vi "LS Durability Main (FPGA).vi"() -> ()   [LabVIEW 2018]
uses:
  <vilib>/rvi/Emulation/niFpgaGetClockAttributes.vi
  <vilib>/rvi/Emulation/niFpgaSctlEmulationGetInTimedLoop.vi
  <vilib>/rvi/Emulation/niFpgaEmulationReportErrorSimple.vi
  <vilib>/rvi/Emulation/niFpgaProcessEmulError.vi
  <vilib>/rvi/eio/common/nirviEmuTemplateMethod_errors.vi
  <vilib>/rvi/Emulation/niFpgaCriticalErrorInLSC.vi
  <vilib>/rvi/DataTransferAndStorage/Container/Common/niFpgaContainerExecOnDevCompGetState.vi
  <vilib>/rvi/Emulation/niFpgaEmulationIsFPGAContextNoSignature.vi
  <vilib>/rvi/errors/niFpgaSetErrorForExecOnDevCompSimple.vi
  <vilib>/rvi/eio/common/nirviEmuReportErrorAndStop.vi
  <vilib>/rvi/DataTransferAndStorage/Container/Common/niFpgaContainerGetUniqueNameForEmu.vi
  <vilib>/rvi/FIFO/Fifo_Resource/nirvififoEmulationSetSize.vi
  <vilib>/rvi/FIFO/Fifo_Resource/nirviFifoEmulationQueueMgr.vi
  <instcachedir>/0/nirviFifoEmulationQueueMgr_E5CAEC123FF24DC58D834DCA3CDAA9B5.lvgen/nirviFifoEmulationQueueMgr_E5CAEC123FF24DC58D834DCA3CDAA9B5_003.vi
  <vilib>/rvi/FIFO/Fifo_Resource/nirvififoEmulationDetermineInputValidOut.vi
  <vilib>/rvi/FIFO/Fifo_Resource/nirvififoEmulationCreateLock.vi
  <vilib>/rvi/FIFO/Fifo_Resource/nirvififoEmulationObtainLock.vi
  <vilib>/rvi/FIFO/Fifo_Resource/nirvififoEmulationReleaseLock.vi
  <vilib>/rvi/occurrence/nirviWaitOnOccurrenceBase.vi
  <vilib>/rvi/errors/nirviReportUnexpectedCaseInternalError.vi
  <vilib>/rvi/errors/nirviReportUnexpectedCaseInternalError (U32).vi
  <vilib>/Utility/error.llb/Clear Errors.vi
  <vilib>/rvi/interface/RandomDataEmulation/niFpgaRandomDataHandleErrors.vi
  <vilib>/eio/EIONode/EIONode.xnode
  <vilib>/rvi/FXPMathLib/FxpAdd/XNode/nifxpmath_Add.xnode
  <vilib>/rvi/DataTransferAndStorage/Container/XNode/niFpgaContainer.xnode
  <vilib>/rvi/FIFO/Fifo_Resource/niFpgaFifoEmulationRefIn.vi
  <vilib>/rvi/FXPMathLib/sim/FxpSim.dll
panel:
  in  "B2offset":fxp<+/-,24,5>
  in  "B1offset":fxp<+/-,24,5>
  out "FIFO microseconds":u32
  in  "V(T)/R(F)":bool=TRUE
  in  "Resistance In":fxp<+/-,28,17>[](array[numeric])=[0.0, 0.0, 0.0, 0.0, 0.0, 0.0, 0.0, 0.0, 0.0, 0.0, 0.0, 0.0]
  out "Anomaly Resamples":fxp<+/-,28,17>[](array[numeric])
  in  "Anomaly Threshold":fxp<+/-,28,17>=0.02978515625
  out "Bank2Active":bool
  out "Bank1Active":bool
  out "Bank2On":bool
  out "Bank1On":bool
  in  "Enable Readings":bool[](array[boolean])=[FALSE, FALSE, FALSE, FALSE, FALSE, FALSE, FALSE, FALSE, FALSE, FALSE, FALSE, FALSE]
  in  "Opens Resets":bool[](array[boolean])=[FALSE, FALSE, FALSE, FALSE, FALSE, FALSE, FALSE, FALSE, FALSE, FALSE, FALSE, FALSE]
  in  "Enable Opens":bool[](array[boolean])=[FALSE, FALSE, FALSE, FALSE, FALSE, FALSE, FALSE, FALSE, FALSE, FALSE, FALSE, FALSE]
  out "Opens Detected":u16[](array[numeric])
  out "Opens Loop Time (usec)":u32=1000
  in  "Bank2(Pulse/Const)":bool
  in  "Bank2Const(On/Off)":bool
  out "Anomalies (Last Cycle)":i32[](array[numeric])
  out "Cycle Starts":bool[](array[boolean])
  out "Anomalies (Total)":i32[](array[numeric])
  out "Anomalies/Cycle":i32[](array[numeric])
  in  "Normal Steps":u32=98
  out "Cycles":u32[](array[numeric])
  out "Anomaly Loop Time (usec)":u32=1000
  out "Steps":u32[](array[numeric])
  in  "Step Threshold":fxp<+/-,28,17>=0.02978515625
  in  "Enable Anomalies":bool[](array[boolean])=[FALSE, FALSE, FALSE, FALSE, FALSE, FALSE, FALSE, FALSE, FALSE, FALSE, FALSE, FALSE]
  in  "Anomaly Resets":bool[](array[boolean])=[FALSE, FALSE, FALSE, FALSE, FALSE, FALSE, FALSE, FALSE, FALSE, FALSE, FALSE, FALSE]
  in  "Bank1Const(On/Off)":bool
  in  "Bank1(Pulse/Const)":bool
  in  "PWM Period (Ticks)":u32=4000000
  in  "Duty (Ticks)":i32=2000000
  in  "Invert PWM?":bool=TRUE
  in  "Cycle Resets":bool[](array[boolean])=[FALSE, FALSE, FALSE, FALSE, FALSE, FALSE, FALSE, FALSE, FALSE, FALSE, FALSE, FALSE]
  in  "Points to Avg":i32=20
  in  "Enable Cycles":bool[](array[boolean])=[FALSE, FALSE, FALSE, FALSE, FALSE, FALSE, FALSE, FALSE, FALSE, FALSE, FALSE, FALSE]
  out "Total Cycles":u32[](array[numeric])
  in  "Cycle Threshold":fxp<+/-,28,17>=1.2001953125
  out "Analog Inputs":fxp<+/-,28,17>[](array[numeric])
  out "AI Loop Time (usec)":u32=70
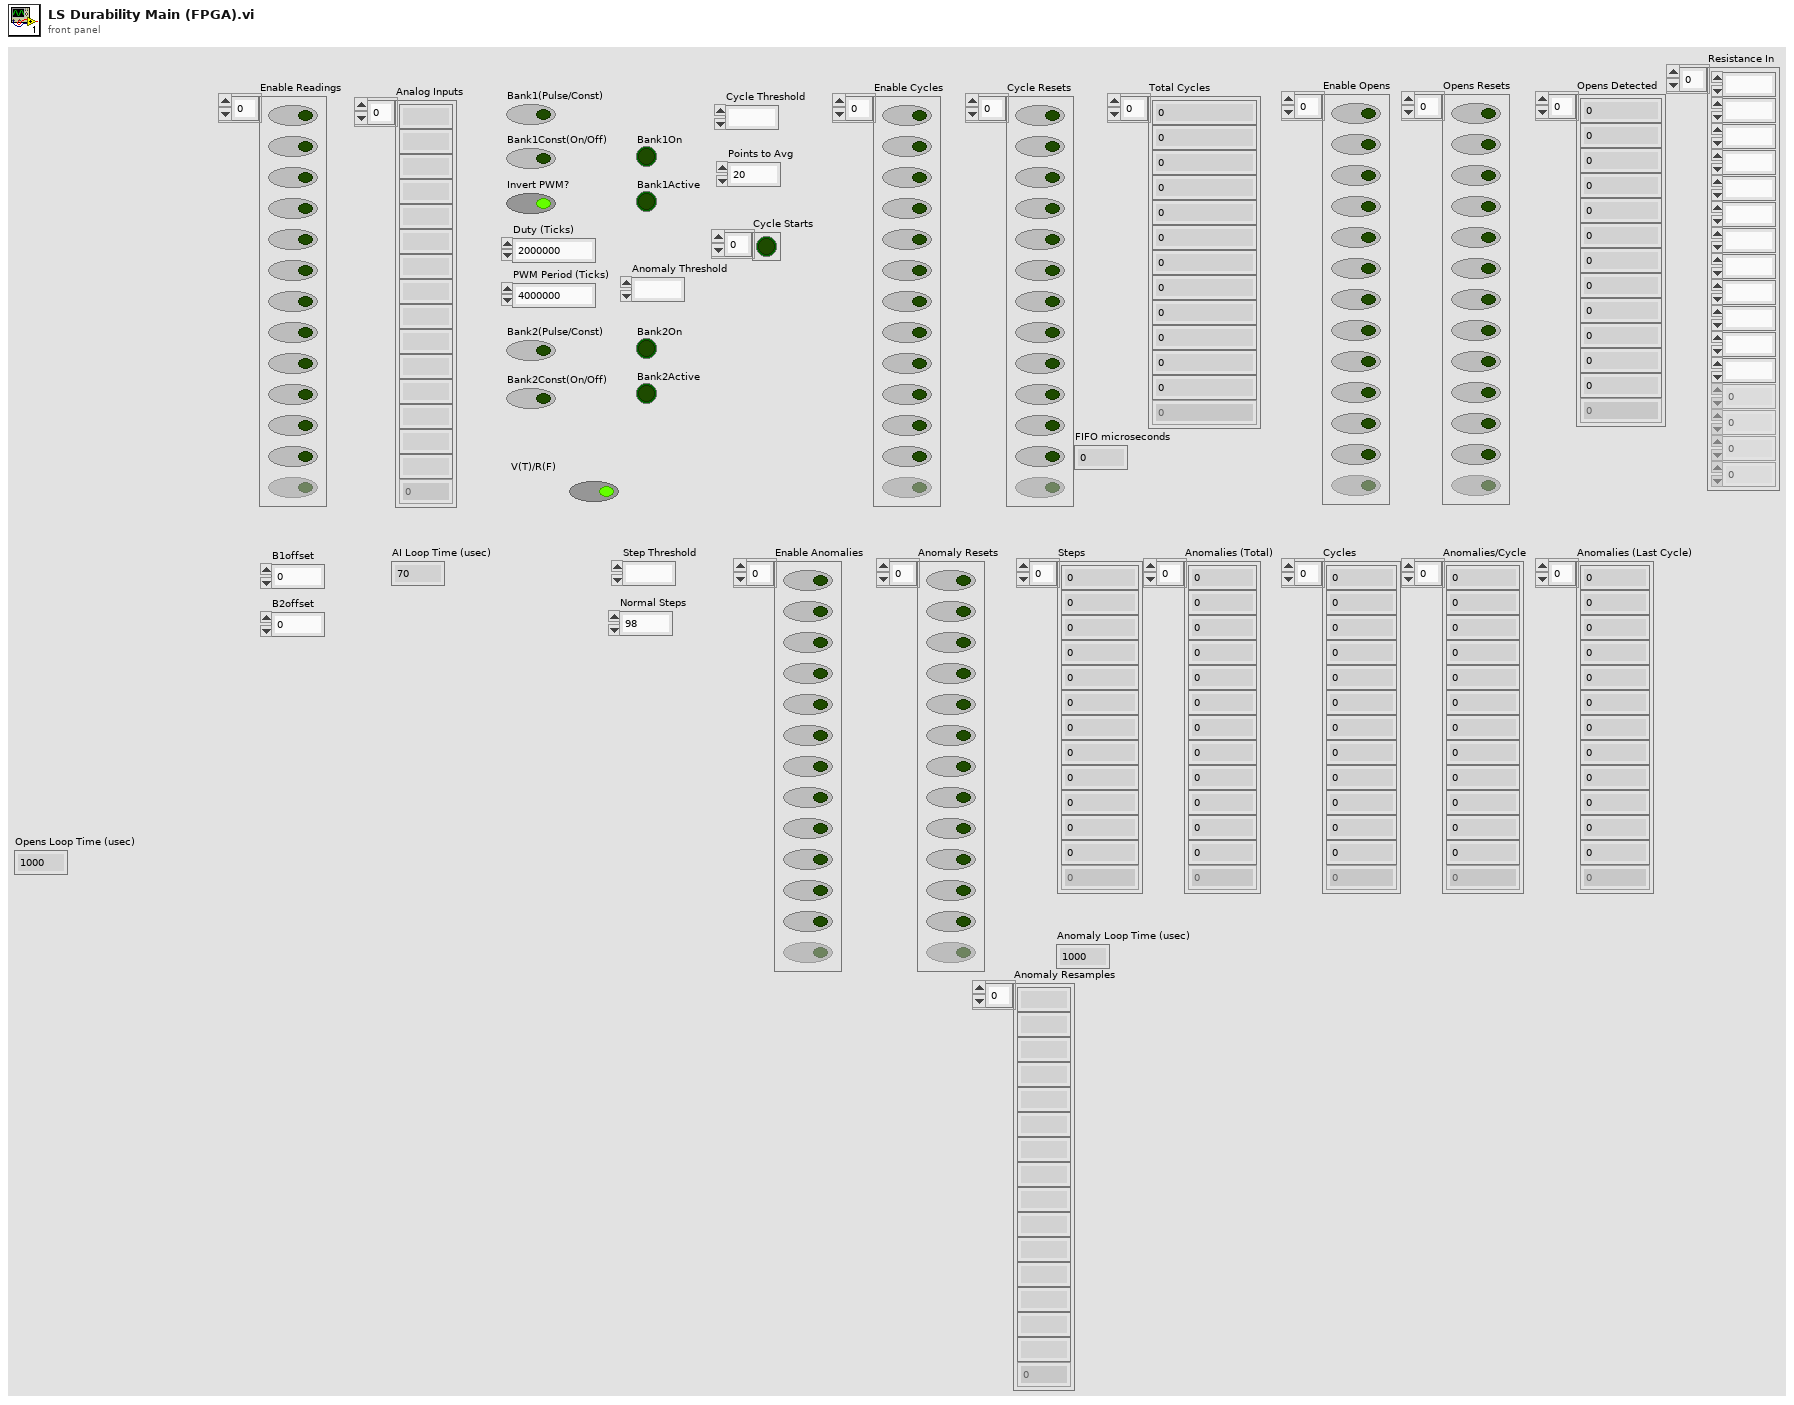
[diagram p1: front panel]
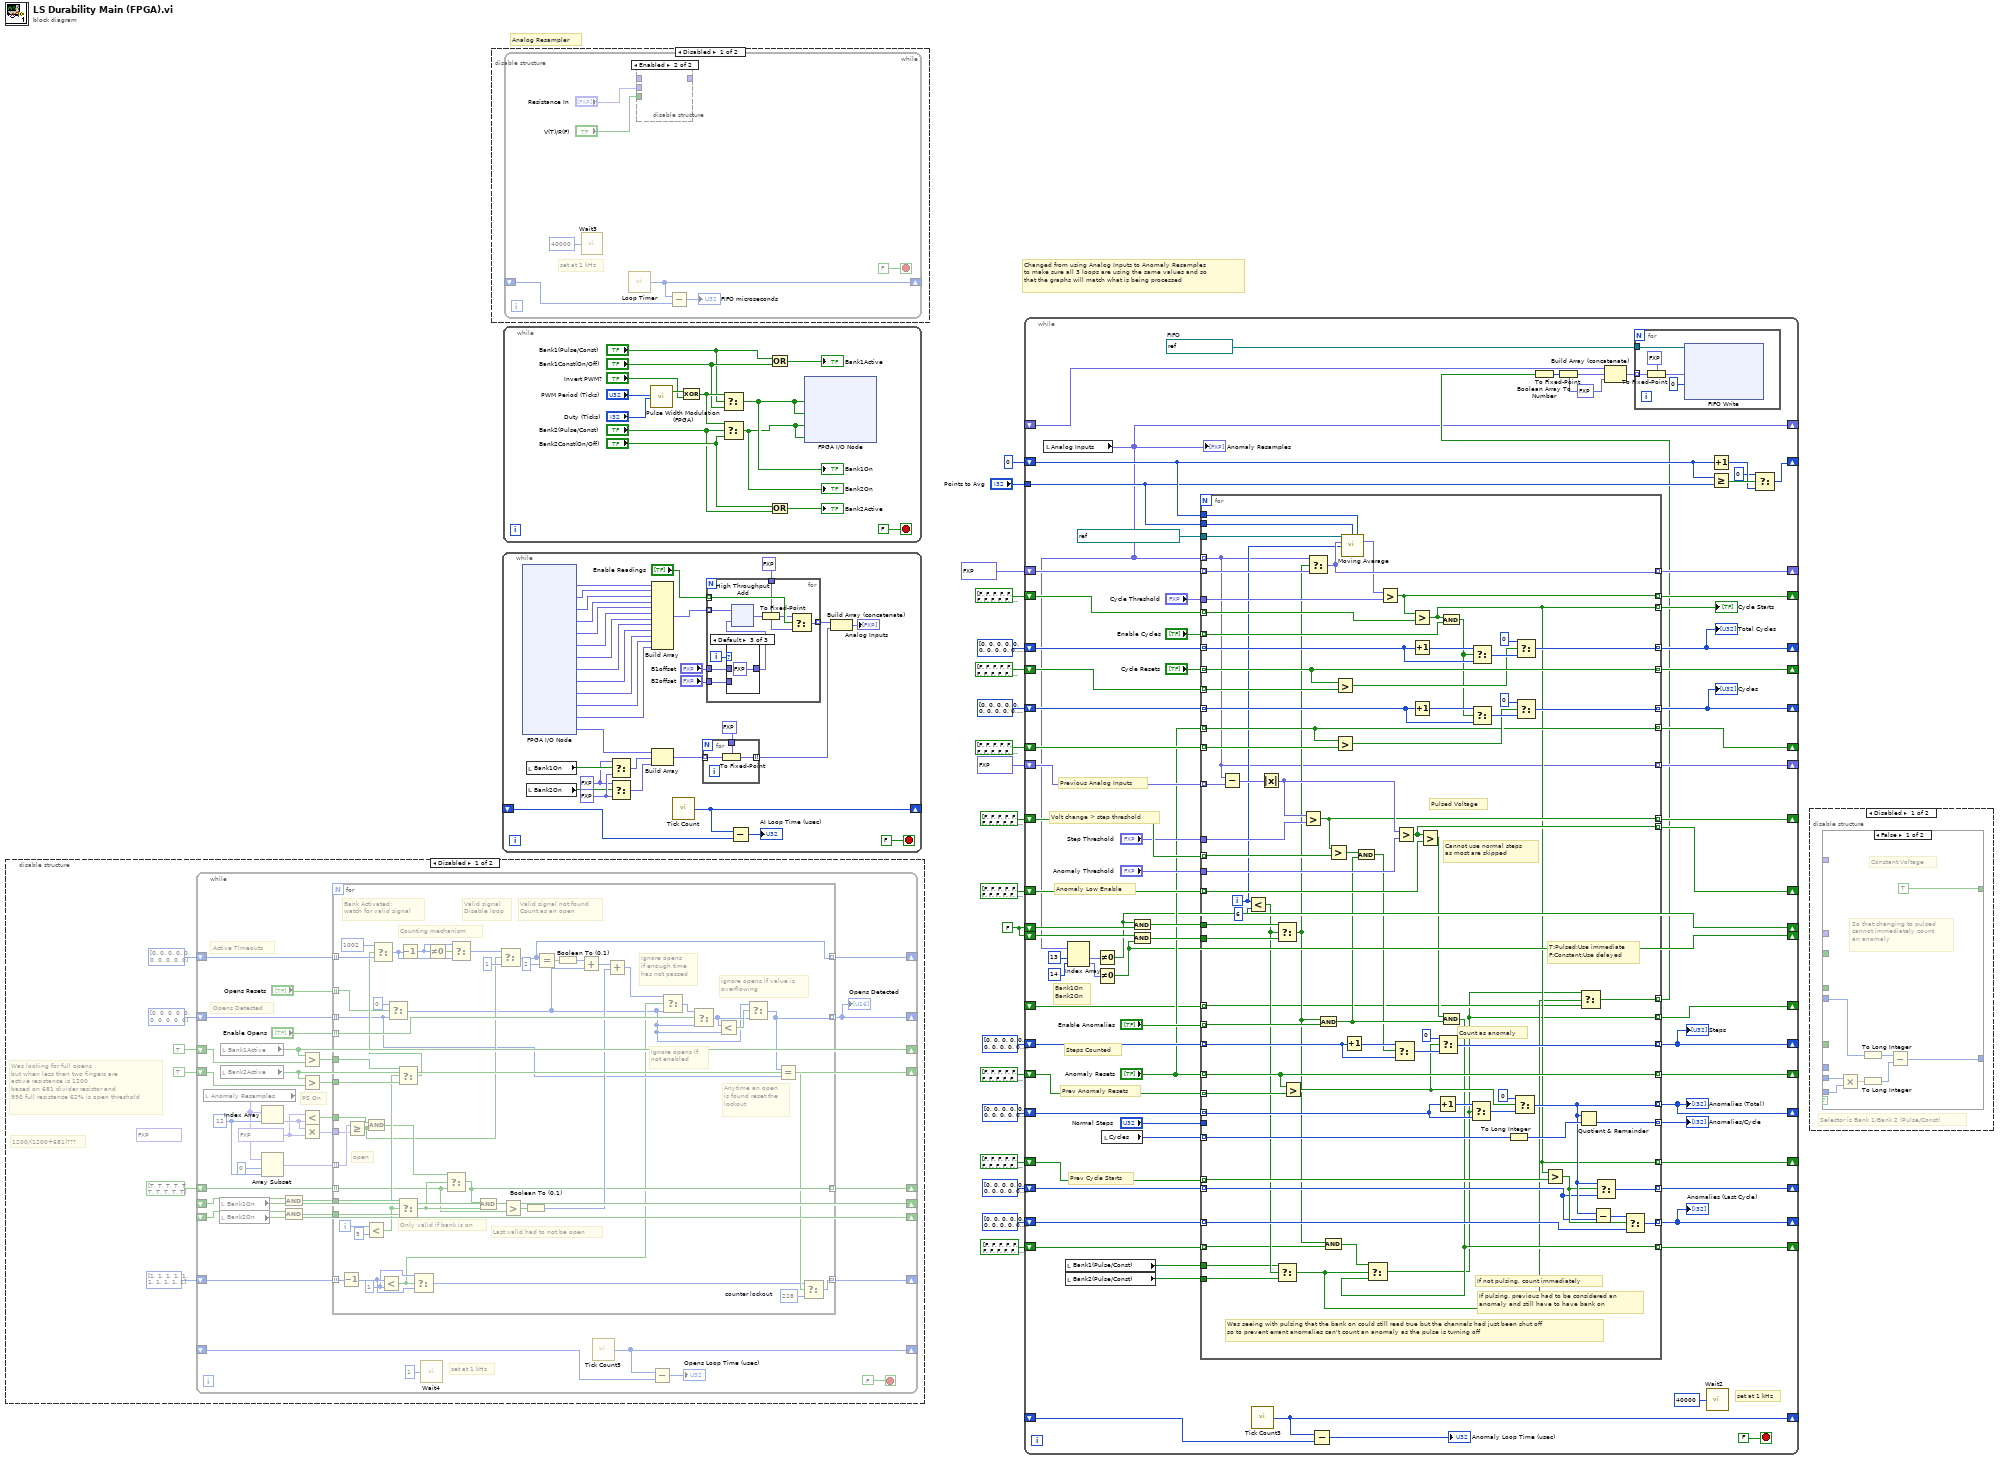
[diagram p0: block diagram]
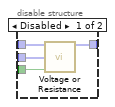
[diagram p2: hidden frame]
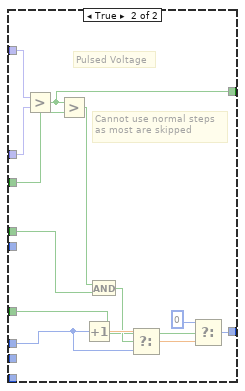
[diagram p5: hidden frame]
diagram:
  w2 = FALSE
  # "Changed from using Analog Inputs to Anomaly Resamples\nto make sure all 3 loops are using the same values and so\nthat the graphs will match what is being processed"
  # "Analog Resampler"
  n1 = disable-structure shown="Disabled" {
    frame Disabled {
      (unwired) fxp<+,8,0> 0.94921875
      # "1200/(1200+681)???"
      # "Was looking for full opens\nbut when less than two fingers are\nactive resistance is 1200\nbased on 681 divider resistor and\n990 full resistance 62% is open threshold"
      n2 = while {
        shift-right: [w58] -> _
        shift-left: _ -> [w57]
        shift-right: [w29] -> _
        shift-left: u8[] [0, 0, 0, 0, 0, 0, 0, 0, 0, 0] -> [w53]
        shift-right: [w38] -> _
        shift-left: u16[] [0, 0, 0, 0, 0, 0, 0, 0, 0, 0] -> [w39]
        shift-right: [w45] -> _
        shift-left: bool[] [TRUE, TRUE, TRUE, TRUE, TRUE, TRUE, TRUE, TRUE, TRUE, TRUE] -> [w44]
        shift-right: [w43] -> _
        shift-left: TRUE ("Bank2Active") -> [w41]
        shift-right: [w42] -> _
        shift-left: TRUE ("Bank1Active") -> [w40]
        shift-right: [w32] -> _
        shift-left: _ -> [w30]
        shift-right: [w33] -> _
        shift-left: _ -> [w31]
        shift-right: [w27] -> _
        shift-left: u16[] [1, 1, 1, 1, 1, 1, 1, 1, 1, 1] -> [w28]
        stop <- FALSE stop-if-true
        w46 = fxp<+,8,0> 0.62109375
        w55 = 12 ("length")
        # "Opens Detected"
        # "Active Timeouts"
        # "PS On"
        # "set at 1 kHz"
        n3 = local read "Anomaly Resamples"() -> (w26:fxp<+/-,28,17>[])
        n4 = local read "Bank1On"() -> (w33:bool)
        n5 = local read "Bank2On"() -> (w32:bool)
        n6 = local read "Bank1Active"() -> (w42:bool)
        n7 = local read "Bank2Active"() -> (w43:bool)
        n8 = Index Array(array=w26, index=w55) -> (element=w47:fxp<+/-,28,17>)
        n9 = Array Subset(array=w26, index=0, length=w55) -> (w48:fxp<+/-,28,17>[])
        n10 = And(x=w31, y=w33) -> (x .and. y?=w35:bool)
        n11 = And(x=w30, y=w32) -> (x .and. y?=w34:bool)
        n12 = Greater?(x=w42, y=w40) -> (0:w52:bool)
        n13 = Greater?(x=w43, y=w41) -> (0:w51:bool)
        n14 = Less?(x=w46, y=w47) -> (x < y?=w50:bool)
        n15 = Multiply(x=w47, y=w46) -> (x*y=w49:fxp<+/-,36,17>)
        n16 = for {
          tunnel: w35 -> [w107]
          tunnel: w34 -> [w106]
          tunnel: w52 -> [w104]
          tunnel: w51 -> [w105]
          tunnel: w53 -> [w65] mode=indexing
          tunnel: w39 -> [w92] mode=indexing
          tunnel: "Opens Resets" -> [w76] mode=indexing
          tunnel: "Enable Opens" -> [w90] mode=indexing
          tunnel: [w66] -> w29 mode=indexing
          tunnel: w49 -> [w87]
          tunnel: w48 -> [w88] mode=indexing
          tunnel: w50 -> [w86]
          tunnel: [w77] -> w45 mode=indexing
          tunnel: w44 -> [w82] mode=indexing
          tunnel: [w80] -> w38 mode=indexing
          tunnel: w28 -> [w71] mode=indexing
          tunnel: [w67] -> w27 mode=indexing
          i -> [w109]
          w68 = u16 228  # counter lockout
          w72 = u16 1 ("y")
          # "Ignore opens if\nnot enabled"
          # "Ignore opens\nif enough time\nhas not passed"
          # "Anytime an open\nis found reset the\nlockout"
          # "ignore opens if value is\noverflowing"
          # "Last valid had to not be open"
          # "Only valid if bank is on"
          # "open"
          # "Valid signal not found\nCount as an open"
          # "Valid signal\nDisable loop"
          # "Counting mechanism"
          # "Bank Activated:\nwatch for valid signal"
          n17 = Decrement(x=w71) -> (x-1=w73:u16)
          n18 = Greater Or Equal?(x=w88, y=w87) -> (x >= y?=w79:bool)
          n19 = Less?(x=w109, y=5) -> (x < y?=w103:bool)
          n20 = And(x=w86, y=w79) -> (x .and. y?=w85:bool)
          n21 = Less?(x=w73, y=w72) -> (x < y?=w62:bool)
          n22 = Select(t=u16 0, s=w76, f=w65) -> (s? t:f=w61:u16)
          n23 = Select(t=w104, s=w103, f=w105) -> (s? t:f=w89:bool)
          n24 = Select(t=u16 1002, s=w89, f=w92) -> (s? t:f=w91:u16)
          n25 = Select(t=w107, s=w103, f=w106) -> (s? t:f=w84:bool)
          n26 = Decrement(x=w91) -> (x-1=w96:u16)
          n27 = Select(t=w72, s=w62, f=w73) -> (s? t:f=w69:u16)
          n28 = Not Equal To 0?(x=w96) -> (x != 0?=w95:bool)
          n29 = Select(t=w85, s=w84, f=w82) -> (s? t:f=w77:bool)
          n30 = Select(t=w96, s=w95, f=w91) -> (s? t:f=w97:u16)
          n31 = And(x=w77, y=w84) -> (x .and. y?=w78:bool)
          n32 = Select(t=w97, s=w79, f=u16 1) -> (s? t:f=w80:u16)
          n33 = Greater?(x=w78, y=w82) -> (0:w83:bool)
          n34 = Boolean To (0,1)(Boolean=w83) -> (0, 1=w81:i16)
          n35 = Equal?(x=w80, y=u16 2) -> (x = y?=w99:bool)
          n36 = Boolean To (0,1)(Boolean=w99) -> (0, 1=w100:i16)
          n37 = Add(x=w100, y=w61) -> (x+y=w101:u16)
          n38 = Add(x=w101, y=w81) -> (x+y=w63:u16)
          n39 = Select(t=w63, s=w62, f=w61) -> (s? t:f=w64:u16)
          n40 = Select(t=w64, s=w90, f=w61) -> (s? t:f=w74:u16)
          n41 = Less?(x=w74, y=w61) -> (x < y?=w75:bool)
          n42 = Select(t=w61, s=w75, f=w74) -> (s? t:f=w66:u16)
          n43 = Equal?(x=w66, y=w65) -> (x = y?=w70:bool)
          n44 = Select(t=w69, s=w70, f=w68) -> (s? t:f=w67:u16)
        }
        "Opens Detected" <- w29
        n45 = call "Wait4"("Count(mSec)"=u32 1) -> ()  [unwired: 1 out]
        n46 = call "Tick Count5"() -> ("Tick Count(uSec)"=w58:u32)
        n47 = Subtract(x=w58, y=w57) -> (x-y=→"Opens Loop Time (usec)":u32)
      }
    }
    frame Enabled {
    }
  }
  n48 = disable-structure shown="Disabled" {
    frame Disabled {
      n49 = while {
        shift-right: [w111] -> _
        shift-left: _ -> [w112]
        stop <- FALSE stop-if-true
        # "set at 1 kHz"
        n50 = call "Wait3"("Count(Ticks)"=u32 40000 ("Count(mSec)")) -> ()  [unwired: 1 out]
        n51 = call "Loop Timer"() -> ("Tick Count(uSec)"=w111:u32)  [unwired: 1 in]
        n52 = disable-structure shown="Enabled" {
          disable-tunnel: _ -> [w120 _]
          disable-tunnel: [w119 _] -> _
          disable-tunnel: "Resistance In" -> [w118 _]
          disable-tunnel: "V(T)/R(F)" -> [w117 _]
          frame Disabled {
            n53 = call "Voltage or Resistance.vi"("Data In"=w120, "Resistance In"=w118, "V(T)/R(F)"=w117) -> ("Data Out"=w119:fxp<+/-,28,17>[])  [unwired: 12 in]
          }
          frame Enabled {
          }
        }
        n54 = Subtract(x=w111, y=w112) -> (x-y=→"FIFO microseconds":u32)
      }
    }
    frame Enabled {
    }
  }
  n55 = while {
    shift-right: [w152] -> _
    shift-left: _ -> [w151]
    stop <- FALSE stop-if-true
    w128 = fxp<+/-,24,5> 1.0 ("AI13")
    w131 = fxp<+/-,24,5> 0.0 ("AI13")
    n56 = xnode "FPGA I/O Node"() -> ("AI0"=w149:fxp<+/-,24,5>, "AI1"=w148:fxp<+/-,24,5>, "AI2"=w147:fxp<+/-,24,5>, "AI3"=w146:fxp<+/-,24,5>, "AI4"=w145:fxp<+/-,24,5>, "AI5"=w121:fxp<+/-,24,5>, "AI6"=w144:fxp<+/-,24,5>, "AI7"=w143:fxp<+/-,24,5>, "AI8"=w142:fxp<+/-,24,5>, "AI9"=w141:fxp<+/-,24,5>, "AI10"=w123:fxp<+/-,24,5>, "AI11"=w122:fxp<+/-,24,5>, "AI12"=w138:fxp<+/-,24,5>)  [unwired: 13 in, 13 out]
    n57 = local read "Bank1On"() -> (w130:bool)
    n58 = local read "Bank2On"() -> (w129:bool)
    n59 = Select(t=w128, s=w130, f=w131) -> (s? t:f=w127:fxp<+/-,24,5>)
    n60 = Select(t=w128, s=w129, f=w131) -> (s? t:f=w126:fxp<+/-,24,5>)
    n61 = Build Array(w149, w148, w147, w146, w145, w121, w144, w143, w142, w141, w123, w122) -> (w140:fxp<+/-,24,5>[])
    n62 = Build Array(w138, w127, w126) -> (w136:fxp<+/-,24,5>[])
    n63 = call "Tick Count"() -> ("Tick Count(uSec)"=w152:u32)
    n64 = for {
      tunnel: w136 -> [w156] mode=indexing
      tunnel: fxp<+/-,28,17> 0.0 ("AI0") -> [w155]
      tunnel: [w154] -> w135 mode=indexing
      n65 = To Fixed-Point(fixed-point type=w155, number=w156) -> (fixed-point=w154:fxp<+/-,28,17>)
    }
    n66 = for {
      tunnel: w140 -> [w159] mode=indexing
      tunnel: fxp<+/-,28,17> 0.0 ("AI0") -> [w164]
      tunnel: [w163] -> w134 mode=indexing
      tunnel: "Enable Readings" -> [w166] mode=indexing
      tunnel: "B1offset" -> [w161]
      tunnel: "B2offset" -> [w160]
      i -> [w162]
      n67 = case shown="Default" w162 {
        tunnel: w161 -> [w167 _ _]
        tunnel: w160 -> [_ w168 _]
        tunnel: [w167 w168 fxp<+/-,24,5> 0.0 ("B2offset")] -> w158
        frame 0..4 {
        }
        frame 5..9 {
        }
        frame Default {
        }
      }
      n68 = xnode "High Throughput Add"("x"=w159, "y"=w158) -> ("x+y"=w157:fxp<+/-,25,6>)
      n69 = To Fixed-Point(fixed-point type=w164, number=w157) -> (fixed-point=w165:fxp<+/-,28,17>)
      n70 = Select(t=w165, s=w166, f=w164) -> (s? t:f=w163:fxp<+/-,28,17>)
    }
    n71 = Subtract(x=w152, y=w151) -> (x-y=→"AI Loop Time (usec)":u32)
    n72 = Build Array (concatenate)(w134, w135) -> (→"Analog Inputs":fxp<+/-,28,17>[])
  }
  n73 = while {
    stop <- FALSE stop-if-true
    n74 = call "Pulse Width Modulation (FPGA).vi"("PWM Period (Ticks)"="PWM Period (Ticks)", "PWM Duty Cycle (Ticks)"="Duty (Ticks)") -> ("PWM DO"=w180:bool)  [unwired: 14 in, 3 out]
    n75 = Exclusive Or(1:"Invert PWM?", 2:w180) -> (0:w178:bool)
    n76 = Select(t=w178, s="Bank1(Pulse/Const)", f="Bank1Const(On/Off)") -> (s? t:f=w171:bool)
    "Bank1On" <- w171
    n77 = Select(t=w178, s="Bank2(Pulse/Const)", f="Bank2Const(On/Off)") -> (s? t:f=w170:bool)
    "Bank2On" <- w170
    n78 = Or(x="Bank1(Pulse/Const)", y="Bank1Const(On/Off)") -> (x .or. y?=→"Bank1Active":bool)
    n79 = Or(x="Bank2Const(On/Off)", y="Bank2(Pulse/Const)") -> (x .or. y?=→"Bank2Active":bool)
    n80 = xnode "FPGA I/O Node"("RMC/DIO0"=w171, "DIO0"=w171, "RMC/DIO1"=w170, "DIO1"=w170) -> ()  [unwired: 5 in, 5 out]
  }
  n81 = while {
    shift-right: [w257] -> _
    shift-left: _ -> [w256]
    shift-right: [w250] -> _
    shift-left: bool[] [FALSE, FALSE, FALSE, FALSE, FALSE, FALSE, FALSE, FALSE, FALSE, FALSE, FALSE, FALSE] -> [w249]
    shift-right: [w247] -> _
    shift-left: u32[] [0, 0, 0, 0, 0, 0, 0, 0, 0, 0, 0, 0] -> [w246]
    shift-right: [w245] -> _
    shift-left: bool[] [FALSE, FALSE, FALSE, FALSE, FALSE, FALSE, FALSE, FALSE, FALSE, FALSE, FALSE, FALSE] -> [w243]
    shift-right: [w252] -> _
    shift-left: fxp<+/-,28,17>[] [0.0, 0.0, 0.0, 0.0, 0.0, 0.0, 0.0, 0.0, 0.0, 0.0, 0.0, 0.0] -> [w251]
    shift-right: [w241] -> _
    shift-left: bool[] [FALSE, FALSE, FALSE, FALSE, FALSE, FALSE, FALSE, FALSE, FALSE, FALSE, FALSE, FALSE] -> [w240]
    shift-right: [w239] -> _
    shift-left: i32[] [0, 0, 0, 0, 0, 0, 0, 0, 0, 0, 0, 0] -> [w237]
    shift-right: [w238] -> _
    shift-left: i32[] [0, 0, 0, 0, 0, 0, 0, 0, 0, 0, 0, 0] -> [w236]
    shift-right: [w193] -> _
    shift-right: [w194] -> _
    shift-right: [w235] -> _
    shift-left: i32[] [0, 0, 0, 0, 0, 0, 0, 0, 0, 0, 0, 0] -> [w234]
    shift-right: [w231] -> _
    shift-left: bool[] [FALSE, FALSE, FALSE, FALSE, FALSE, FALSE, FALSE, FALSE, FALSE, FALSE, FALSE, FALSE] -> [w232]
    shift-left: w2 -> [w229]
    shift-left: w2 -> [w230]
    tunnel: "Points to Avg" -> [w204]
    shift-right: [w224] -> _
    shift-left: 0 ("Moving Point Index") -> [w205]
    shift-right: [w206] -> _
    shift-left: fxp<+/-,28,17>[] [0.0, 0.0, 0.0, 0.0, 0.0, 0.0, 0.0, 0.0, 0.0, 0.0, 0.0, 0.0] ("Analog Inputs") -> [w208]
    shift-right: [w209] -> _
    shift-left: bool[] [FALSE, FALSE, FALSE, FALSE, FALSE, FALSE, FALSE, FALSE, FALSE, FALSE, FALSE, FALSE] -> [w211]
    shift-right: [w214] -> _
    shift-left: u32[] [0, 0, 0, 0, 0, 0, 0, 0, 0, 0, 0, 0] -> [w215]
    shift-right: [w216] -> _
    shift-left: bool[] [FALSE, FALSE, FALSE, FALSE, FALSE, FALSE, FALSE, FALSE, FALSE, FALSE, FALSE, FALSE] -> [w218]
    shift-right: [w220] -> _
    shift-left: u32[] [0, 0, 0, 0, 0, 0, 0, 0, 0, 0, 0, 0] -> [w221]
    shift-right: [w219] -> _
    shift-left: bool[] [FALSE, FALSE, FALSE, FALSE, FALSE, FALSE, FALSE, FALSE, FALSE, FALSE, FALSE, FALSE] -> [w223]
    shift-right: [w200] -> _
    shift-left: bool[] [FALSE, FALSE, FALSE, FALSE, FALSE, FALSE, FALSE, FALSE, FALSE, FALSE, FALSE, FALSE] -> [w199]
    shift-right: [w184] -> _
    shift-left: _ -> [w188]
    shift-right: [w186] -> _
    shift-left: _ -> [w187]
    stop <- FALSE stop-if-true
    w189 = refnum<k21> "Analog Data"  # FIFO
    w191 = fxp<+/-,28,17> -15.0 ("AI0")
    # "Bank1On\nBank2On"
    # "Anomaly Low Enable"
    # "Prev Cycle Starts"
    # "Prev Anomaly Resets"
    # "Steps Counted"
    # "Volt change > step threshold"
    # "Previous Analog Inputs"
    # "set at 1 kHz"
    n82 = local read "Analog Inputs"() -> (w184:fxp<+/-,28,17>[])
    "Anomaly Resamples" <- w184
    n83 = local read "Bank1(Pulse/Const)"() -> (w202:bool)
    n84 = local read "Bank2(Pulse/Const)"() -> (w201:bool)
    n85 = Index Array(array=w184, index #1=13 ("index"), index #2=14 ("index")) -> (element #1=w196:fxp<+/-,28,17>, element #2=w195:fxp<+/-,28,17>)
    n86 = Not Equal To 0?(x=w196) -> (x != 0?=w193:bool)
    n87 = Not Equal To 0?(x=w195) -> (x != 0?=w194:bool)
    n88 = local read "Cycles"() -> (w242:u32[])
    n89 = And(x=w193, y=w230) -> (x .and. y?=w254:bool)
    n90 = And(x=w229, y=w194) -> (x .and. y?=w253:bool)
    n91 = for {
      tunnel: [w309] -> w250 mode=indexing
      tunnel: w249 -> [w324] mode=indexing
      tunnel: w246 -> [w318] mode=indexing
      tunnel: [w317] -> w247 mode=indexing
      tunnel: "Step Threshold" -> [w310]
      tunnel: "Enable Anomalies" -> [w280] mode=indexing
      tunnel: "Anomaly Resets" -> [w326] mode=indexing
      tunnel: [w326] -> w245 mode=indexing
      tunnel: w243 -> [w327] mode=indexing
      tunnel: [w270] -> w252 mode=indexing
      tunnel: w251 -> [w341] mode=indexing
      tunnel: "Normal Steps" -> [_]
      tunnel: w242 -> [w333] mode=indexing
      tunnel: [w332] -> w244 mode=indexing
      tunnel: [w334] -> w235 mode=indexing
      tunnel: [w278] -> w241 mode=indexing
      tunnel: w240 -> [w329] mode=indexing
      tunnel: [w331] -> w239 mode=indexing
      tunnel: w237 -> [w316] mode=indexing
      tunnel: [w330] -> w238 mode=indexing
      tunnel: w236 -> [w315] mode=indexing
      tunnel: w254 -> [w346]
      tunnel: w253 -> [w345]
      tunnel: w234 -> [w343] mode=indexing
      tunnel: "Anomaly Threshold" -> [w339]
      tunnel: w232 -> [w338] mode=indexing
      tunnel: [w337] -> w231 mode=indexing
      tunnel: w223 -> [w308] mode=indexing
      tunnel: "Anomaly Resets" -> [w301] mode=indexing
      tunnel: w221 -> [w304] mode=indexing
      tunnel: [w303] -> w220 mode=indexing
      tunnel: [w301] -> w219 mode=indexing
      tunnel: w218 -> [w300] mode=indexing
      tunnel: "Cycle Resets" -> [w299] mode=indexing
      tunnel: [w299] -> w216 mode=indexing
      tunnel: w215 -> [w294] mode=indexing
      tunnel: [w293] -> w214 mode=indexing
      tunnel: "Enable Cycles" -> [w292] mode=indexing
      tunnel: "Cycle Threshold" -> [w289]
      tunnel: w211 -> [w290] mode=indexing
      tunnel: [w278] -> w210 mode=indexing
      tunnel: [w288] -> w209 mode=indexing
      tunnel: w208 -> [w287] mode=indexing
      tunnel: w184 -> [w270] mode=indexing
      tunnel: refnum<k21> "Running Avg Memory" ("Memory") -> [w286]
      tunnel: [w285] -> w206 mode=indexing
      tunnel: w205 -> [w283]
      tunnel: w204 -> [w282]
      tunnel: w202 -> [w276]
      tunnel: w201 -> [w275]
      tunnel: [w274] -> w200 mode=indexing
      tunnel: w199 -> [w272] mode=indexing
      tunnel: [w266] -> w186 mode=indexing
      tunnel: w187 -> [w268] mode=indexing
      tunnel: [w267] -> w185 mode=indexing
      i -> [w284]
      # "T:Pulsed:Use immediate\nF:Constant:Use delayed"
      # "If pulsing, previous had to be considered an\nanomaly and still have to have bank on"
      # "If not pulsing, count immediately"
      # "Count as anomaly"
      # "Was seeing with pulsing that the bank on could still read true but the channels had just been shut off\nso to prevent errant anomalies can't count an anomaly as the pulse is turning off"
      # "Cannot use normal steps\nas most are skipped"
      # "Pulsed Voltage"
      n92 = Subtract(x=w270, y=w341) -> (x-y=w342:fxp<+/-,29,18>)
      n93 = Less?(x=w284, y=6) -> (x < y?=w277:bool)
      n94 = Absolute Value(x=w342) -> (abs(x)=w340:fxp<+,28,17>)
      n95 = Select(t=w346, s=w277, f=w345) -> (s? t:f=w273:bool)
      n96 = Select(t=w276, s=w277, f=w275) -> (s? t:f=w269:bool)
      n97 = Greater?(x=w326, y=w327) -> (0:w319:bool)
      n98 = Greater?(x=w340, y=w310) -> (0:w309:bool)
      n99 = Select(t=w270, s=w273, f=w287) -> (s? t:f=w285:fxp<+/-,28,17>)
      n100 = And(x=w273, y=w280) -> (x .and. y?=w323:bool)
      n101 = And(x=w273, y=w272) -> (x .and. y?=w271:bool)
      n102 = Greater?(x=w309, y=w324) -> (0:w325:bool)
      n103 = Greater?(x=w299, y=w300) -> (0:w295:bool)
      n104 = Greater?(x=w301, y=w308) -> (0:w302:bool)
      n105 = call "Moving Average.vi"("Memory In"=w286, "N (# of Ave Pts 127 max)"=w282, "Moving Point Index"=w283, "Data IN"=w285, "Channel#"=w284) -> ("Averaged Data"=w281:fxp<+/-,28,17>)  [unwired: 10 in]
      n106 = Increment(x=w318) -> (x+1=w320:u32)
      n107 = And(x=w325, y=w323) -> (x .and. y?=w279:bool)
      n108 = Greater?(x=w281, y=w289) -> (0:w288:bool)
      n109 = Select(t=w320, s=w279, f=w318) -> (s? t:f=w321:u32)
      n110 = Greater?(x=w340, y=w339) -> (0:w337:bool)
      n111 = Greater?(x=w288, y=w290) -> (0:w278:bool)
      n112 = Increment(x=w294) -> (x+1=w296:u32)
      n113 = Increment(x=w304) -> (x+1=w307:u32)
      n114 = Greater?(x=w337, y=w338) -> (0:w311:bool)
      n115 = Increment(x=w343) -> (x+1=w312:i32)
      n116 = Select(t=u32 0, s=w319, f=w321) -> (s? t:f=w317:u32)
      n117 = And(x=w278, y=w292) -> (x .and. y?=w291:bool)
      n118 = And(x=w311, y=w323) -> (x .and. y?=w274:bool)
      n119 = Select(t=w271, s=w269, f=w274) -> (s? t:f=w266:bool)
      n120 = Select(t=w312, s=w266, f=w343) -> (s? t:f=w313:i32)
      n121 = Select(t=w296, s=w291, f=w294) -> (s? t:f=w297:u32)
      n122 = Select(t=w307, s=w291, f=w304) -> (s? t:f=w306:u32)
      n123 = To Long Integer(number=w333) -> (32bit integer=w335:i32)
      n124 = Select(t=0, s=w319, f=w313) -> (s? t:f=w334:i32)
      n125 = Select(t=u32 0, s=w295, f=w297) -> (s? t:f=w293:u32)
      n126 = Select(t=u32 0, s=w302, f=w306) -> (s? t:f=w303:u32)
      n127 = Greater?(x=w278, y=w329) -> (0:w328:bool)
      n128 = Quotient & Remainder(x=w334, y=w335) -> (floor(x/y)=w332:i32)  [unwired: 1 out]
      n129 = Select(t=w266, s=w269, f=w268) -> (s? t:f=w267:bool)
      n130 = Subtract(x=w334, y=w316) -> (x-y=w336:i32)
      n131 = Select(t=w334, s=w328, f=w316) -> (s? t:f=w331:i32)
      n132 = Select(t=w336, s=w328, f=w315) -> (s? t:f=w330:i32)
    }
    "Steps" <- w247
    "Anomalies/Cycle" <- w244
    "Anomalies (Total)" <- w235
    "Anomalies (Last Cycle)" <- w238
    "Total Cycles" <- w214
    "Cycles" <- w220
    "Cycle Starts" <- w210
    n133 = call "Tick Count3"() -> ("Tick Count(uSec)"=w257:u32)
    n134 = Subtract(x=w257, y=w256) -> (x-y=→"Anomaly Loop Time (usec)":u32)
    n135 = Boolean Array To Number(Boolean array=w185) -> (number=w192:u16)
    n136 = To Fixed-Point(fixed-point type=w191, number=w192) -> (fixed-point=w190:fxp<+/-,28,17>)
    n137 = Build Array (concatenate)(w188, w190, w191) -> (w203:fxp<+/-,28,17>[])
    n138 = for {
      tunnel: w189 -> [w265]
      tunnel: w203 -> [w264] mode=indexing
      n139 = To Fixed-Point(fixed-point type=fxp<+/-,22,11> 0.0 ("AI0"), number=w264) -> (fixed-point=w263:fxp<+/-,22,11>)
      n140 = xnode ("FIFO Write")("Element"=w263, "Timeout"=0, "FIFO In"=w265) -> ()  [unwired: 2 out]
    }
    n141 = call "Wait2"("Count(Ticks)"=u32 40000 ("Count(mSec)")) -> ()  [unwired: 1 out]
    n142 = Increment(x=w205) -> (x+1=w226:i32)
    n143 = Greater Or Equal?(x=w205, y=w204) -> (x >= y?=w227:bool)
    n144 = Select(t=0, s=w227, f=w226) -> (s? t:f=w224:i32)
  }
  n145 = disable-structure shown="Disabled" {
    frame Disabled {
      # "Selector is Bank 1/Bank 2 (Pulse/Const)"
      n146 = case shown="False" {
        selector: _ -> [_ _]
        tunnel: _ -> [w354 _]
        tunnel: _ -> [w350 _]
        tunnel: [w349 w363] -> _
        tunnel: _ -> [w347 _]
        tunnel: _ -> [_ w364]
        tunnel: _ -> [_ w360]
        tunnel: _ -> [_ w361]
        tunnel: _ -> [_ w359]
        tunnel: _ -> [_ w358]
        tunnel: [TRUE w357] -> _
        tunnel: _ -> [_ w355]
        frame False {
          # "So that changing to pulsed\ncannot immediately count\nan anomaly"
          # "Constant Voltage"
          n147 = Multiply(x=w354, y=w350) -> (x*y=w353:dbl)
          n148 = To Long Integer(number=w347) -> (32bit integer=w352:i32)
          n149 = To Long Integer(number=w353) -> (32bit integer=w351:i32)
          n150 = Subtract(x=w352, y=w351) -> (x-y=w349:i32)
        }
        frame True {
          # "Cannot use normal steps\nas most are skipped"
          # "Pulsed Voltage"
          n151 = Greater?(x=w360, y=w359) -> (0:w357:bool)
          n152 = Greater?(x=w357, y=w358) -> (0:w356:bool)
          n153 = Increment(x=w364) -> (x+1=w365:dbl)
          n154 = And(x=w356, y=w361) -> (x .and. y?=w362:bool)
          n155 = Select(t=w365, s=w362, f=w364) -> (s? t:f=w366:dbl)
          n156 = Select(t=0, s=w355, f=w366) -> (s? t:f=w363:i32)
        }
      }
    }
    frame Enabled {
    }
  }
